vi "instantiate_vectorstore_destinationconnector.vi"(0 "abstract_vector_base":refnum<class "abstract_vector_base.lvclass">, 5 "store_id":string, 11 "error in (no error)":errorcluster) -> (4 "destination_vectorstore out":refnum<class "destination_vectorstore.lvclass">, 15 "error out":errorcluster)   [LabVIEW 2020, in "destination_vectorstore.lvclass"]
uses:
  destination_vectorstore.lvclass
  vectorstore/abstract_vector_base/abstract_vector_base.lvclass
  destination_vectorstore.lvclass/destination_vectorstore.ctl
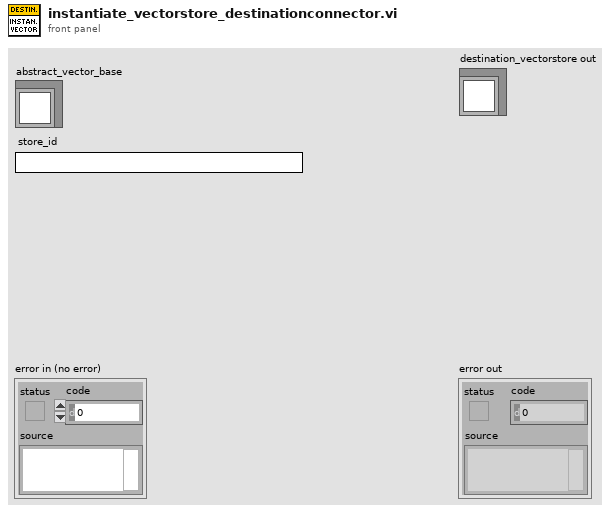
[diagram p1: front panel]
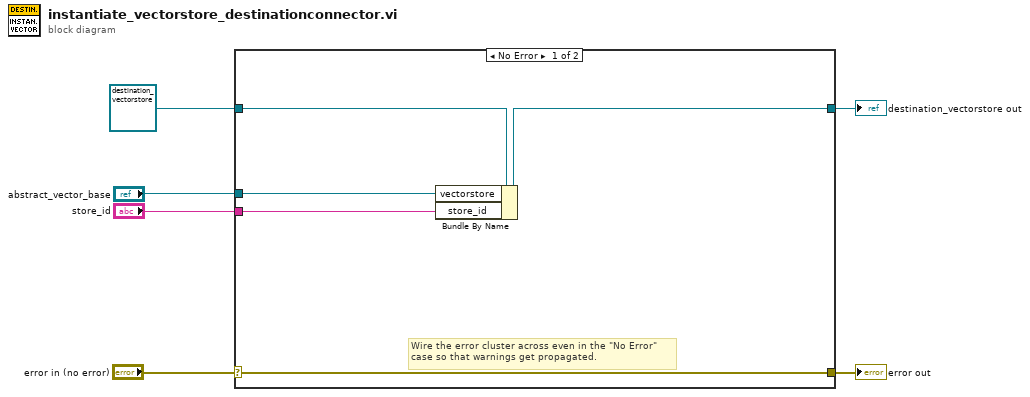
[diagram p0: block diagram]
diagram:
  n1 = case shown="No Error" "error in (no error)" {
    selector: "error in (no error)" -> [w11 w13]
    tunnel: [w11 w13] -> w5
    tunnel: [w9 w12] -> w3
    tunnel: refnum<class "destination_vectorstore.lvclass"> refnum ("destination_vectorstore in") -> [w10 w12]
    tunnel: "abstract_vector_base" -> [w8 _]
    tunnel: "store_id" -> [w7 _]
    frame No Error {
      # "Wire the error cluster across even in the \"No Error\"\ncase so that warnings get propagated."
      n2 = Bundle By Name(cluster=w10, "vectorstore"=w8, "store_id"=w7) -> (w9:refnum<class "destination_vectorstore.lvclass">)
    }
    frame Error {
    }
  }
  "error out" <- w5
  "destination_vectorstore out" <- w3
